vi "execute.vi"(8 "error in (no error)":errorcluster caption="错误输入（无错误）", 11 "Task 2 in":refnum<class "Task2.lvclass">) -> (0 "error out":errorcluster caption="错误输出", 3 "Task 2 out":refnum<class "Task2.lvclass">)   [LabVIEW 2024, in "Task2.lvclass"]
doc: "本VI是为《我和LabVIEW》一书编写的示例。\n关于本书的介绍请参考网页：\nhttp://ruanqizhen.spaces.live.com/blog/cns!5852D4F797C53FB6!4310.entry"
uses:
  Task2.lvclass
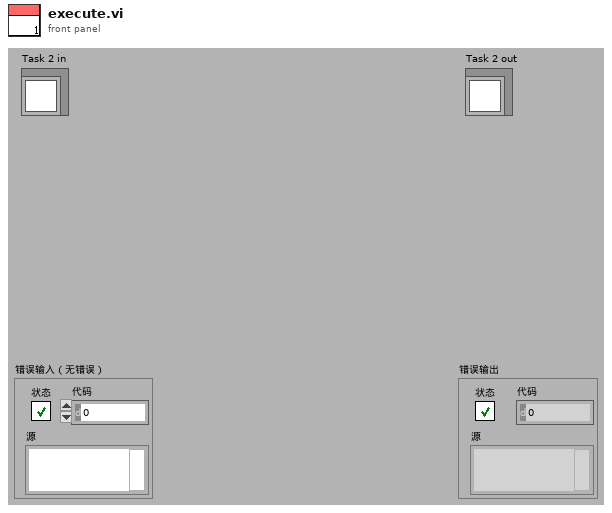
[diagram p1: front panel]
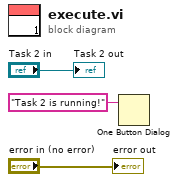
[diagram p0: block diagram]
diagram:
  n1 = One Button Dialog(message="Task 2 is running!" ("消息")) -> ()  [unwired: 2 out]
  "error out" <- "error in (no error)"
  "Task 2 out" <- "Task 2 in"
